vi "Add Serial Device Channel.vi"(4 "Property Values":variant[](array[variant]), 5 "Override Default Channel?":bool, 6 "Property names":string[](array[string]), 7 "Extra Page GUID":string="03D3BB99-1485-13A6-561D1F898F032919", 8 "에러 입력(에러 없음)":errorcluster, 9 "Channel":T1, 10 "Channel Name":string, 11 "Device Item Ref In":T3 format="%.0x") -> (0 "에러 출력":errorcluster, 3 "Device Item Ref Out":T3 format="%.0x")   [LabVIEW 2017, in "Serial Communcation Devices Custom Device.lvlib"]
uses:
  Serial Communcation Devices Custom Device.lvlib
  <vilib>/NI Veristand/Custom Device API/Custom Device Item Ref.ctl
  <vilib>/NI Veristand/Custom Device API/Custom Device Channel.ctl
  <vilib>/NI Veristand/Custom Device API/Custom Device Channel Type.ctl
  <vilib>/NI Veristand/Custom Device API/Custom Device API.lvlib
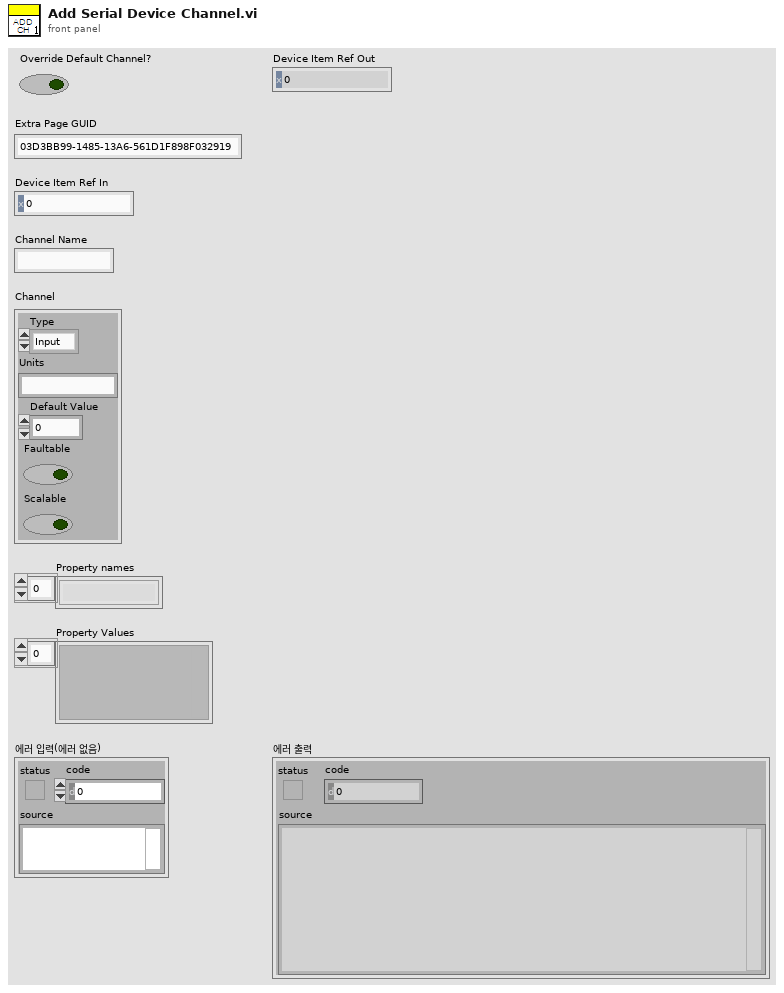
[diagram p1: front panel]
types:
  T1 = typedef "Custom Device API.lvlib/Custom Device Channel.ctl" = cluster{"Type":T2, "Units":string, "Default Value":dbl, "Faultable":bool, "Scalable":bool}
  T2 = typedef "Custom Device API.lvlib/Custom Device Channel Type.ctl" = enum16{"Input", "Output"}
  T3 = typedef "Custom Device API.lvlib/Custom Device Item Ref.ctl" = u64
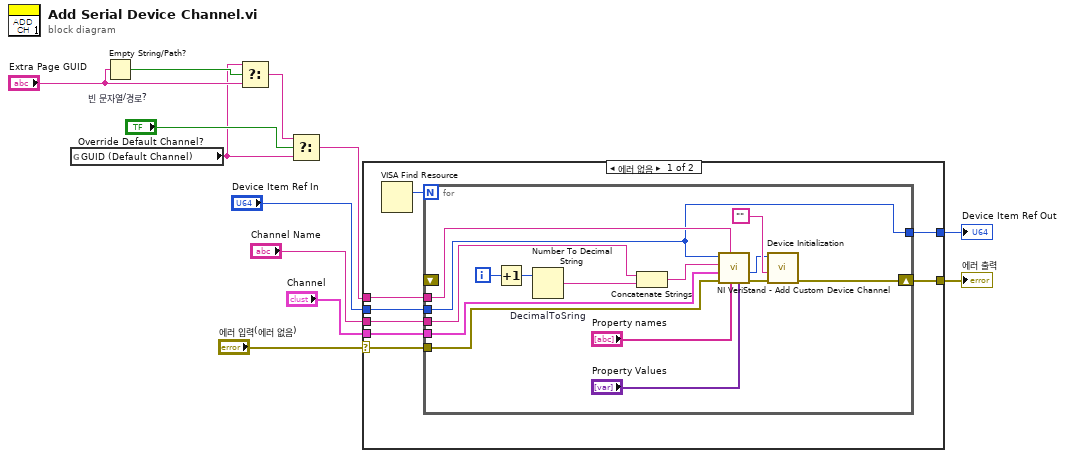
[diagram p0: block diagram]
diagram:
  n1 = global read "글로벌 1.vi" "GUID (Default Channel)"() -> (w1:string)
  n2 = Empty String/Path? "빈 문자열/경로?"(string/path="Extra Page GUID") -> (empty?=w3:bool)
  n3 = Select(t=w1, s=w3, f="Extra Page GUID") -> (s? t:f=w5:string)
  n4 = Select(t=w5, s="Override Default Channel?", f=w1) -> (s? t:f=w4:string)
  n5 = case shown="에러 없음" "에러 입력(에러 없음)" {
    selector: "에러 입력(에러 없음)" -> [w18 w37]
    tunnel: [w16 w37] -> w7
    tunnel: [w17 w36] -> w8
    tunnel: "Device Item Ref In" -> [w14 w36]
    tunnel: "Channel Name" -> [w15 _]
    tunnel: "Channel" -> [w19 _]
    tunnel: w4 -> [w13 _]
    frame No Error {
      n6 = VISA Find Resource() -> (2:w20:u32)  [unwired: 3 in, 2 out]
      n7 = for {
        N: w20 -> [_]
        tunnel: w19 -> [w35]
        tunnel: w18 -> [w32]
        tunnel: [w23] -> w17
        shift-right: [w24] -> w16
        shift-left: _ -> [_]
        tunnel: w15 -> [w28]
        tunnel: w14 -> [w23]
        tunnel: w13 -> [w26]
        i -> [w30]
        n8 = Increment(x=w30) -> (x+1=w29:i32)
        n9 = Number To Decimal String "DecimalToSring"(number=w29) -> (decimal integer string=w31:string)  [unwired: 1 in]
        n10 = Concatenate Strings(w28, w31) -> (w27:string)
        n11 = call <vilib>:"NI VeriStand - Add Custom Device Channel.vi"("Property Values"="Property Values", "Property names"="Property names", "GUID (Default Channel)"=w26, "error in (no error)"=w32, "Channel"=w35, "Channel Name"=w27, "Parent Ref in"=w23) -> ("error out"=w25:errorcluster, "Channel Ref"=w21:T3)  [unwired: 1 in, 2 out]
        n12 = call "Device Initialization.vi"("에러 입력(에러 없음)"=w25, "VISA Resource Name"="", "Channel Ref"=w21) -> ("에러 출력"=w24:errorcluster)  [unwired: 8 in]
      }
    }
    frame Error {
    }
  }
  "Device Item Ref Out" <- w8
  "에러 출력" <- w7
